vi "main.vi"() -> ()   [LabVIEW 2021]
uses:
  C:/Users/Rainy/Desktop/labviewPdfToWord/dll/ClassLibraryLabview.dll
  dll/ClassLibraryLabview.dll
panel:
  in  "word 路径":path
  in  "pdf路径":path
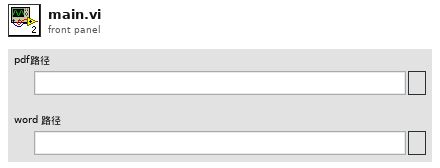
[diagram p1: front panel]
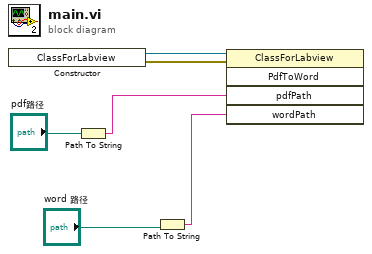
[diagram p0: block diagram]
diagram:
  n1 = constructor class="ClassForLabview"() -> (reference out=w6:refnum<k24>, error out=w5:errorcluster)  [unwired: 3 in, 1 out]
  n2 = Path To String(path="pdf路径") -> (string=w2:string)
  n3 = Path To String(path="word 路径") -> (string=w3:string)
  n4 = invoke on="调用节点" class="ClassForLabview" method="PdfToWord"(reference=w6, error in=w5, "pdfPath"=w2, "wordPath"=w3) -> ()  [unwired: 1 in, 5 out]
